vi "GetProperties.vi"(8 "error in":errorcluster, 11 "Cluster in":refnum<class "Cluster.lvclass">) -> (0 "error out":errorcluster, 3 "Cluster out":refnum<class "Cluster.lvclass">)   [LabVIEW 2014, in "Raspberry Pi Compatible Compiler for LabVIEW.lvlib" / "Cluster.lvclass"]
uses:
  Cluster.lvclass
  Cluster.lvclass/Cluster.ctl
  Control/Control.lvclass
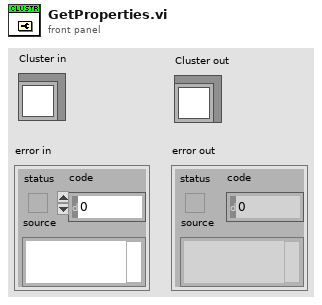
[diagram p1: front panel]
types:
  T1 = typedef "LVBoundsTypeDef.ctl" = cluster{"Width":u32, "Height":u32}
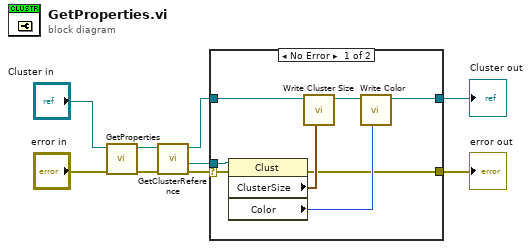
[diagram p0: block diagram]
diagram:
  n1 = call-parent "GetProperties.vi"("error in"="error in", "Control in"="Cluster in") -> ("error out"=w6:errorcluster, "Control out"=w7:refnum<class "Cluster.lvclass">)  [unwired: 8 in]
  n2 = call "GetClusterReference.vi"("error in"=w6, "Cluster in"=w7) -> ("error out"=w5:errorcluster, "cluster reference"=w4:refnum<vi>, "Cluster out"=w3:refnum<class "Cluster.lvclass">)  [unwired: 7 in]
  n3 = case shown="No Error" w5 {
    selector: w5 -> [w17 w18]
    tunnel: w4 -> [w16 _]
    tunnel: w3 -> [w15 w19]
    tunnel: [w11 w19] -> w2
    tunnel: [w10 w18] -> w1
    frame No Error {
      n4 = property class="Clust"(reference=w16, error in=w17) -> (error out=w10:errorcluster, "ClusterSize"=w14:T1, "Color"=w12:u32)  [unwired: 1 out]
      n5 = call "Write Cluster Size.vi"("Cluster Size"=w14, "Cluster in"=w15) -> ("Cluster out"=w13:refnum<class "Cluster.lvclass">)  [unwired: 7 in]
      n6 = call "Write Color.vi"("Color"=w12, "Cluster in"=w13) -> ("Cluster out"=w11:refnum<class "Cluster.lvclass">)  [unwired: 7 in]
    }
    frame Error {
    }
  }
  "error out" <- w1
  "Cluster out" <- w2
